vi "Initialize Custom Device Settings.vi"(8 "error in":errorcluster, 10 "Compiled Settings":variant, 11 "Engine Settings in":T2) -> (0 "error out":errorcluster, 1 "ChannelRefs":T1, 3 "Engine Settings out":T2)   [LabVIEW 2026, in "Template.lvlib" / "Template.lvclass"]
uses:
  Template.lvclass
  Types/TargetSettings.ctl
  Template.lvclass/Template.ctl
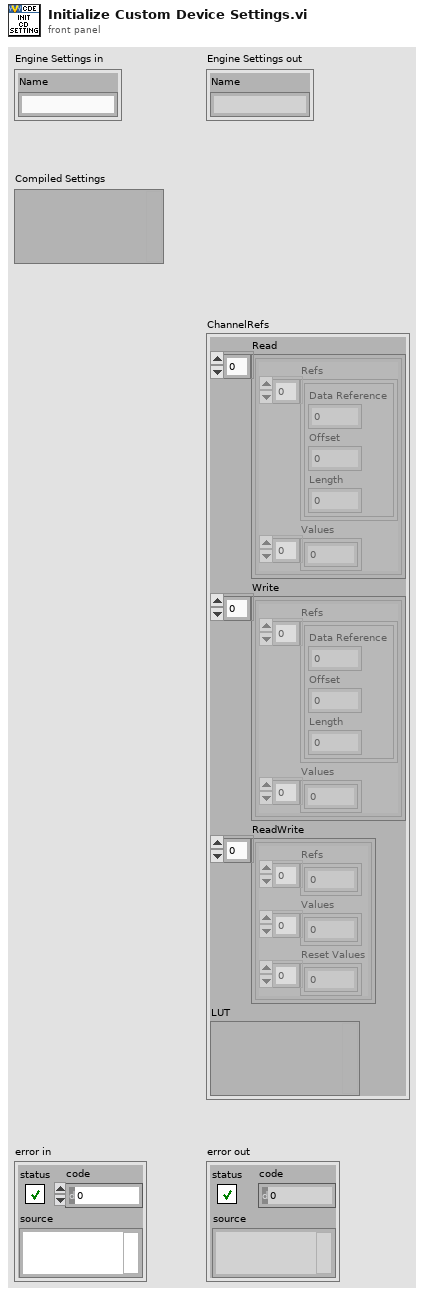
[diagram p1: front panel]
types:
  T1 = cluster{"Read":cluster{"Refs":cluster{"Data Reference":i32, "Offset":u64, "Length":u64}[], "Values":dbl[]}[], "Write":cluster{"Refs":cluster{"Data Reference":i32, "Offset":u64, "Length":u64}[], "Values":dbl[]}[], "ReadWrite":cluster{"Refs":i32[], "Values":dbl[], "Reset Values":dbl[]}[], "LUT":variant}
  T2 = typedef "Template.lvlib/Template.lvclass/TargetSettings.ctl" = cluster{"Name":string}
  T3 = cluster{cluster{string}, cluster{"Channel Refs":cluster{"Read":cluster{"Refs":cluster{"Data Reference":i32, "Offset":u64, "Length":u64}[], "Values":dbl[]}[], "Write":cluster{"Refs":cluster{"Data Reference":i32, "Offset":u64, "Length":u64}[], "Values":dbl[]}[], "ReadWrite":cluster{"Refs":i32[], "Values":dbl[], "Reset Values":dbl[]}[], "LUT":variant}, "Group Settings":cluster{"Name":string, "Type":enum16{"Output/Write", "Input/Read", "Input/ReadWrite"}, "Channel Settings":cluster{"Name":string, "TypeName":string, "ChannelProperties":variant}[]}[]}}
  T4 = enum16{"Output/Write", "Input/Read", "Input/ReadWrite"}
  T5 = cluster{"Channel Refs":cluster{"Read":cluster{"Refs":cluster{"Data Reference":i32, "Offset":u64, "Length":u64}[], "Values":dbl[]}[], "Write":cluster{"Refs":cluster{"Data Reference":i32, "Offset":u64, "Length":u64}[], "Values":dbl[]}[], "ReadWrite":cluster{"Refs":i32[], "Values":dbl[], "Reset Values":dbl[]}[], "LUT":variant}, "Group Settings":cluster{"Name":string, "Type":enum16{"Output/Write", "Input/Read", "Input/ReadWrite"}, "Channel Settings":cluster{"Name":string, "TypeName":string, "ChannelProperties":variant}[]}[]}
  T6 = cluster{"Name":string, "Type":enum16{"Output/Write", "Input/Read", "Input/ReadWrite"}, "Channel Settings":cluster{"Name":string, "TypeName":string, "ChannelProperties":variant}[]}[]
  T7 = cluster{"Name":string, "TypeName":string, "ChannelProperties":variant}[]
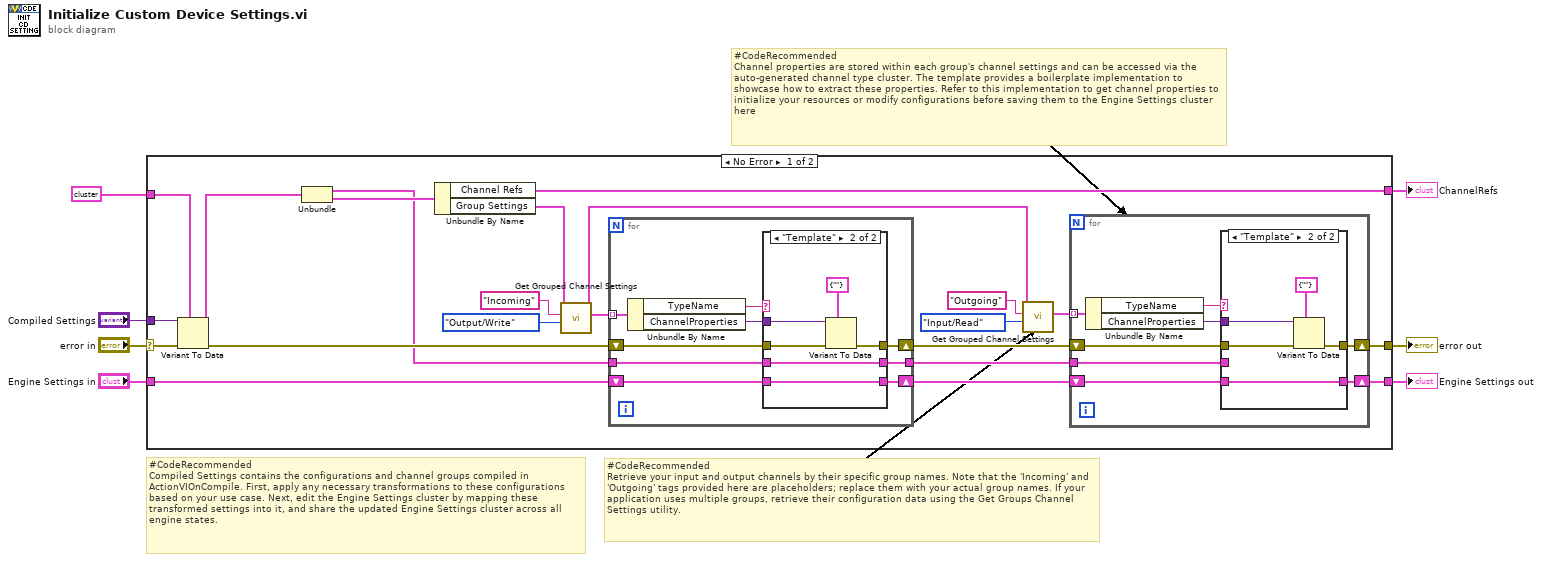
[diagram p0: block diagram]
diagram:
  # "#CodeRecommended\nChannel properties are stored within each group's channel settings and can be accessed via the auto-generated channel type cluster. The template provides a boilerplate implementation to showcase how to extract these properties. Refer to this implementation to get channel properties to initialize your resources or modify configurations before saving them to the Engine Settings cluster here"
  # "#CodeRecommended\nRetrieve your input and output channels by their specific group names. Note that the 'Incoming' and 'Outgoing' tags provided here are placeholders; replace them with your actual group names. If your application uses multiple groups, retrieve their configuration data using the Get Groups Channel Settings utility."
  # "#CodeRecommended\nCompiled Settings contains the configurations and channel groups compiled in ActionVIOnCompile. First, apply any necessary transformations to these configurations based on your use case. Next, edit the Engine Settings cluster by mapping these transformed settings into it, and share the updated Engine Settings cluster across all engine states."
  n1 = case shown="No Error" "error in" {
    selector: "error in" -> [w28 w64]
    tunnel: [w29 w64] -> w6
    tunnel: [w22 w63] -> w5
    tunnel: "Engine Settings in" -> [w23 w63]
    tunnel: "Compiled Settings" -> [w25 _]
    tunnel: [w24 _] -> w2
    tunnel: T3 {{""}, {"Channel Refs"={"Read"=[], "Write"=[], "ReadWrite"=[], "LUT"=variant}, "Group Settings"=[]}} ("CompiledSettings") -> [w21 _]
    frame No Error {
      n2 = Variant To Data(error in=w28, type=w21, Variant=w25) -> (data=w20:T3, error out=w27:errorcluster)
      n3 = Unbundle(w20) -> (w8:cluster{string}, w19:T5)
      n4 = Unbundle By Name(w19) -> ("Channel Refs"=w24:T1, "Group Settings"=w18:T6)
      n5 = call "Get Grouped Channel Settings.vi"("Type"=T4."Output/Write", "Group Name"="Incoming", "Group Settings"=w18) -> ("Channel Settings"=w15:T7, "Name based Group Settings"=w12:T6)  [unwired: 6 in, 1 out]
      n6 = for {
        tunnel: w15 -> [w36] mode=indexing
        tunnel: w8 -> [w33]
        shift-right: [w32] -> w9
        shift-left: w23 -> [w31]
        tunnel: [w30] -> w10
        shift-right: [w37] -> w26
        shift-left: w27 -> [w38]
        n7 = Unbundle By Name(w36) -> ("TypeName"=w35:string, "ChannelProperties"=w34:variant)
        n8 = case "Incoming" shown="\"Template\"" w35 {
          tunnel: w34 -> [_ w42]
          tunnel: w33 -> [w39 w45]
          tunnel: [w40 w44] -> w32
          tunnel: w31 -> [w40 w44]
          tunnel: [w39 w45] -> w30
          tunnel: w38 -> [w41 w46]
          tunnel: [w41 w47] -> w37
          frame Default {
          }
          frame "Template" {
            n9 = Variant To Data(error in=w46, type=cluster{string} {""} ("Properties"), Variant=w42) -> (error out=w47:errorcluster)  [unwired: 1 out]
          }
        }
      }
      n10 = call "Get Grouped Channel Settings.vi"("Type"=T4."Input/Read", "Group Name"="Outgoing", "Group Settings"=w12) -> ("Channel Settings"=w11:T7)  [unwired: 6 in, 2 out]
      n11 = for {
        tunnel: w11 -> [w53] mode=indexing
        tunnel: w10 -> [w50]
        shift-right: [w49] -> w22
        shift-left: w9 -> [w48]
        shift-right: [w54] -> w29
        shift-left: w26 -> [w55]
        n12 = Unbundle By Name(w53) -> ("TypeName"=w52:string, "ChannelProperties"=w51:variant)
        n13 = case "Outgoing" shown="\"Template\"" w52 {
          tunnel: w51 -> [_ w58]
          tunnel: w50 -> [_ _]
          tunnel: [w56 w60] -> w49
          tunnel: w48 -> [w56 w60]
          tunnel: w55 -> [w57 w61]
          tunnel: [w57 w62] -> w54
          frame Default {
          }
          frame "Template" {
            n14 = Variant To Data(error in=w61, type=cluster{string} {""} ("Properties"), Variant=w58) -> (error out=w62:errorcluster)  [unwired: 1 out]
          }
        }
      }
    }
    frame Error {
    }
  }
  "error out" <- w6
  "Engine Settings out" <- w5
  "ChannelRefs" <- w2
